vi "attackTacticCheckStateChange.vi"(8 "error in (no error)":errorcluster, 9 "Robot In":refnum<class "Robot.lvclass">, 10 "Game in":refnum<class "Game.lvclass">, 11 "AttackTacticVSS in":refnum<class "AttackTacticVSS.lvclass">) -> (0 "error out":errorcluster, 2 "State":enum16{"Kick", "Exit", "GoToBall", "BallToGoal"}(ring), 3 "AttackTacticVSS out":refnum<class "AttackTacticVSS.lvclass">)   [LabVIEW 2020, in "AttackTacticVSS.lvclass"]
uses:
  AttackTacticVSS.lvclass
  Game_class/Game.lvclass
  Robot_class/Robot.lvclass
  C:/ROBOIME/SSL_AI/Object_class/Object.lvclass
  Utilities_class/Utilities.lvclass
  Game_class/Game.lvclass/Game.ctl
  Object_class/Object.lvclass/Object.ctl
  Team_class/Team.lvclass/Team.ctl
  Object_class/Read x.vi
  Object_class/Read y.vi
  Game_class/Read BallRef.vi
  Game_class/Read EnemyRef.vi
  Game_class/Read FieldRef.vi
  Team_class/Read RobotRef.vi
  Enemy_class/Enemy.lvclass
  C:/ROBOIME/SSL_AI/Team_class/Team.lvclass
  Ball_class/Ball.lvclass
  Field_class/Field.lvclass
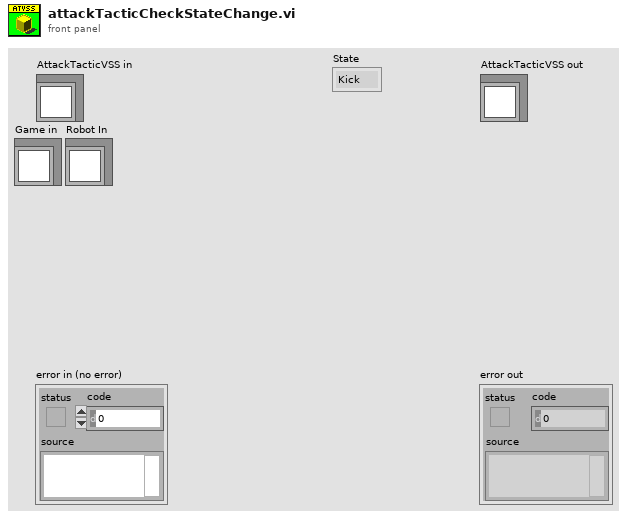
[diagram p1: front panel]
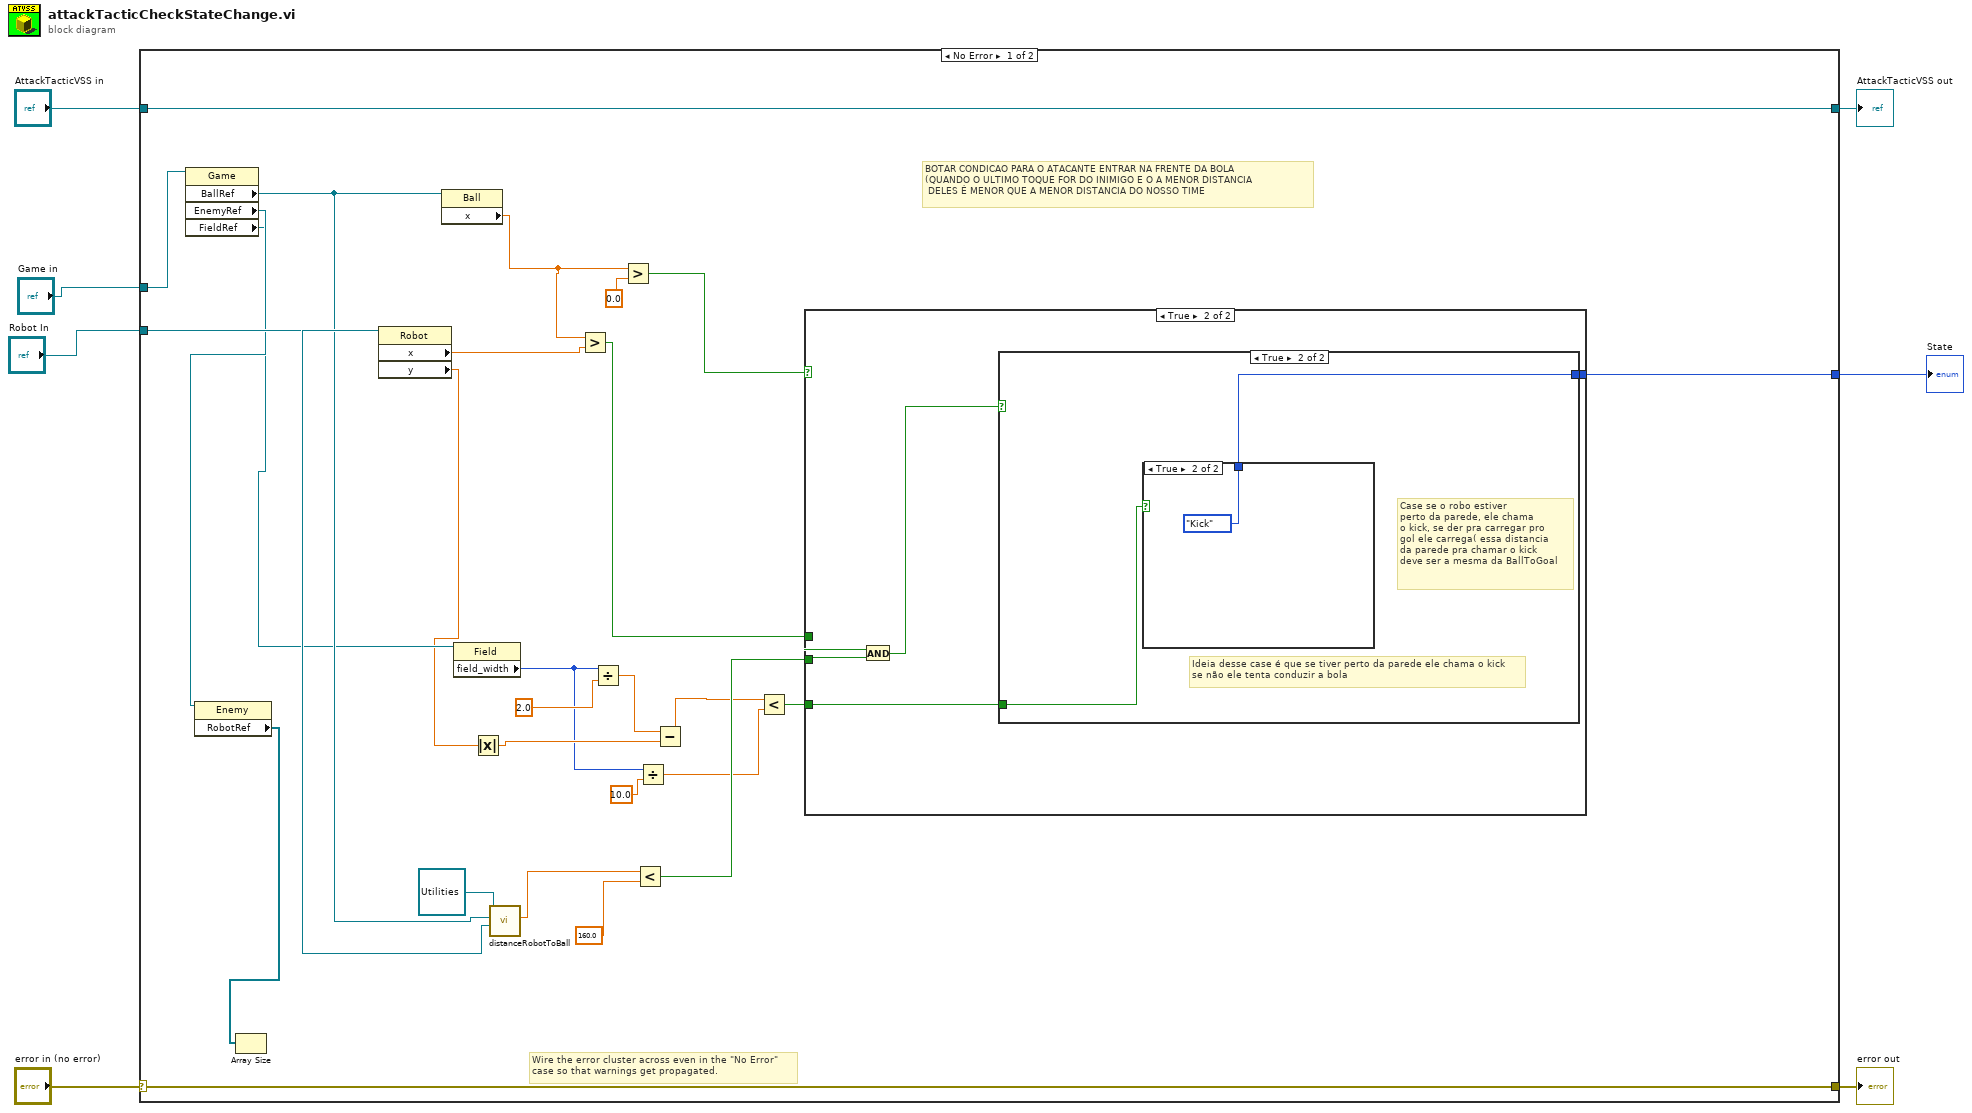
[diagram p0: block diagram]
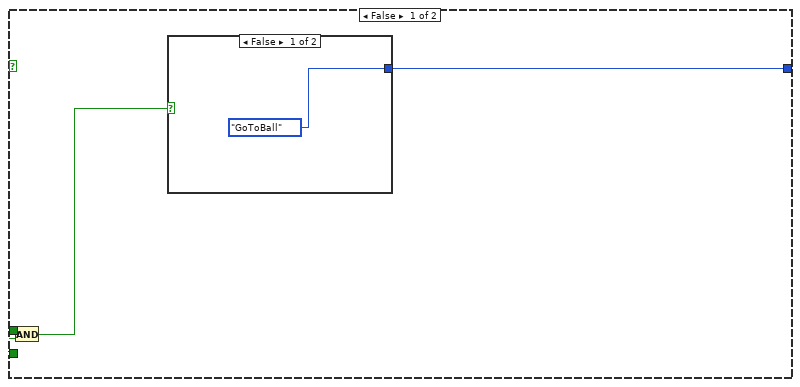
[diagram p2: hidden frame]
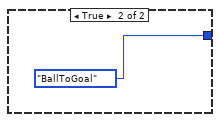
[diagram p3: hidden frame]
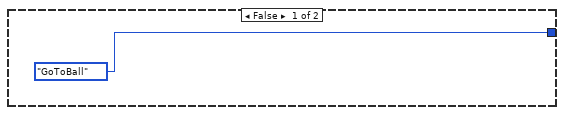
[diagram p4: hidden frame]
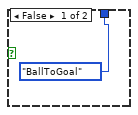
[diagram p5: hidden frame]
diagram:
  n1 = case shown="No Error" "error in (no error)" {
    selector: "error in (no error)" -> [w34 w53]
    tunnel: [w34 w53] -> w6
    tunnel: [w35 w52] -> w4
    tunnel: "AttackTacticVSS in" -> [w35 w52]
    tunnel: "Game in" -> [w33 _]
    tunnel: "Robot In" -> [w30 _]
    tunnel: [w23 _] -> w1
    frame No Error {
      # "BOTAR CONDICAO PARA O ATACANTE ENTRAR NA FRENTE DA BOLA\n(QUANDO O ULTIMO TOQUE FOR DO INIMIGO E O A MENOR DISTANCIA\n DELES É MENOR QUE A MENOR DISTANCIA DO NOSSO TIME"
      # "Wire the error cluster across even in the \"No Error\"\ncase so that warnings get propagated."
      n2 = property class="Game"(reference=w33) -> ("BallRef"=w29:refnum<class "Ball.lvclass">, "EnemyRef"=w20:refnum<class "Enemy.lvclass">, "FieldRef"=w18:refnum<class "Field.lvclass">)  [unwired: 1 in, 2 out]
      n3 = property class="Enemy"(reference=w20) -> ("RobotRef"=w19:refnum<class "Robot.lvclass">[])  [unwired: 1 in, 2 out]
      n4 = Array Size(array=w19) -> ()  [unwired: 1 out]
      n5 = property class="Robot"(reference=w30) -> (reference out=w31:refnum<class "Robot.lvclass">, "x"=w16:dbl, "y"=w11:dbl)  [unwired: 1 in, 1 out]
      n6 = property class="Ball"(reference=w29) -> ("x"=w22:dbl)  [unwired: 1 in, 2 out]
      n7 = property class="Field"(reference=w18) -> ("field_width"=w10:i32)  [unwired: 1 in, 2 out]
      n8 = Absolute Value(x=w11) -> (abs(x)=w14:dbl)
      n9 = call "distanceRobotToBall.vi"("Robot"=w31, "Ball"=w29, "Utilities in"=refnum<class "Utilities.lvclass"> refnum) -> ("Distance Robot To Ball"=w26:dbl)  [unwired: 6 in, 2 out]
      n10 = Greater?(x=w22, y=w16) -> (0:w21:bool)
      n11 = Divide(x=w10, y=2.0) -> (x/y=w15:dbl)
      n12 = Greater?(x=w22, y=0.0) -> (0:w27:bool)
      n13 = Less?(x=w26, y=160.0) -> (x < y?=w24:bool)
      n14 = Divide(x=w10, y=10.0) -> (x/y=w8:dbl)
      n15 = Subtract(x=w15, y=w14) -> (x-y=w13:dbl)
      n16 = Less?(x=w13, y=w8) -> (x < y?=w12:bool)
      n17 = case shown="True" w27 {
        tunnel: w24 -> [w38 w44]
        tunnel: [w39 w46] -> w23
        tunnel: w21 -> [w37 w45]
        tunnel: w12 -> [_ w42]
        frame False {
          n18 = And(x=w37, y=w38) -> (x .and. y?=w36:bool)
          n19 = case shown="False" w36 {
            tunnel: [enum16{"Kick", "Exit", "GoToBall", "BallToGoal"}."GoToBall" ("State") enum16{"Kick", "Exit", "GoToBall", "BallToGoal"}."BallToGoal" ("State")] -> w39
            frame False {
            }
            frame True {
            }
          }
        }
        frame True {
          n20 = And(x=w45, y=w44) -> (x .and. y?=w43:bool)
          n21 = case shown="True" w43 {
            tunnel: [enum16{"Kick", "Exit", "GoToBall", "BallToGoal"}."GoToBall" ("State") w48] -> w46
            tunnel: w42 -> [_ w49]
            frame False {
            }
            frame True {
              # "Ideia desse case é que se tiver perto da parede ele chama o kick\nse não ele tenta conduzir a bola"
              # "Case se o robo estiver\nperto da parede, ele chama\no kick, se der pra carregar pro\ngol ele carrega( essa distancia\nda parede pra chamar o kick\ndeve ser a mesma da BallToGoal"
              n22 = case shown="True" w49 {
                tunnel: [enum16{"Kick", "Exit", "GoToBall", "BallToGoal"}."BallToGoal" ("State") enum16{"Kick", "Exit", "GoToBall", "BallToGoal"}."Kick" ("State")] -> w48
                frame False {
                }
                frame True {
                }
              }
            }
          }
        }
      }
    }
    frame Error {
    }
  }
  "error out" <- w6
  "AttackTacticVSS out" <- w4
  "State" <- w1
